vi "Ctrl.Graph.StyleFont.vi"(8 "error in (no error)":errorcluster, 10 "Font Info":T1, 11 "Graph Ctrl Ref in":refnum<vi>) -> (0 "error out":errorcluster, 3 "Graph Ctrl Ref out":refnum<vi>)   [LabVIEW 2017, in "JKI Simple Localization.lvlib"]
uses:
  API/JKI Simple Localization.lvlib
  Definitions/Private/Font Info -- Cluster.ctl
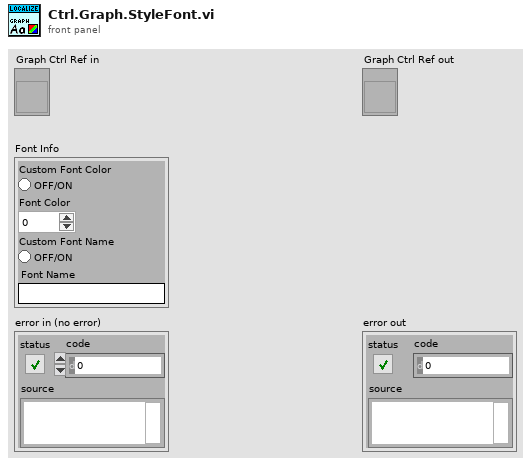
[diagram p1: front panel]
types:
  T1 = typedef "JKI Simple Localization.lvlib/Font Info -- Cluster.ctl" = cluster{"Custom Font Color":bool, "Font Color":u32, "Custom Font Name":bool, "Font Name":string}
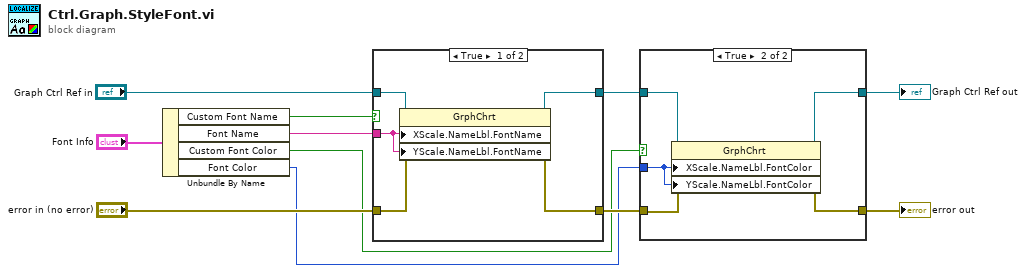
[diagram p0: block diagram]
diagram:
  n1 = Unbundle By Name("Font Info") -> ("Custom Font Name"=w10:bool, "Font Name"=w6:string, "Custom Font Color"=w2:bool, "Font Color"=w1:u32)
  n2 = case shown="True" w10 {
    tunnel: [w14 w18] -> w9
    tunnel: "error in (no error)" -> [w15 w18]
    tunnel: w6 -> [w12 _]
    tunnel: "Graph Ctrl Ref in" -> [w16 w17]
    tunnel: [w13 w17] -> w4
    frame True {
      n3 = property class="GrphChrt"(reference=w16, error in=w15, "XScale.NameLbl.FontName"=w12, "YScale.NameLbl.FontName"=w12) -> (reference out=w13:refnum<vi>, error out=w14:errorcluster)
    }
    frame False {
    }
  }
  n4 = case shown="True" w2 {
    tunnel: w9 -> [w20 w23]
    tunnel: [w20 w22] -> w7
    tunnel: w1 -> [_ w21]
    tunnel: w4 -> [w19 w25]
    tunnel: [w19 w24] -> w3
    frame False {
    }
    frame True {
      n5 = property class="GrphChrt"(reference=w25, error in=w23, "XScale.NameLbl.FontColor"=w21, "YScale.NameLbl.FontColor"=w21) -> (reference out=w24:refnum<vi>, error out=w22:errorcluster)
    }
  }
  "error out" <- w7
  "Graph Ctrl Ref out" <- w3
